vi "Get Protocol Type.vi"(8 "error in (no error)":errorcluster, 11 "RS-xxx to GPIB ConvBox in":refnum<class "RS-xxx to GPIB ConvBox.lvclass">) -> (0 "error out":errorcluster, 2 "Protocol Type":T1=enum."AK RS-XXX", 3 "RS-xxx to GPIB ConvBox out":refnum<class "RS-xxx to GPIB ConvBox.lvclass">)   [LabVIEW 2018, in "Protocols.lvlib" / "RS-xxx to GPIB ConvBox.lvclass"]
doc: "Returns GPIB ConvBox protocol type Enum.\n\nInput:\nRS-xxx to GPIB ConvBox in: represents an instance of the RS-xxx to GPIB ConvBox protocol class.\n\nOutput: \nRS-xxx to GPIB ConvBox out: represents an instance of the RS-xxx to GPIB ConvBox protocol class provided as input.\nProtocol Type: represents the type of the protocol in Enum format."
uses:
  RS-xxx to GPIB ConvBox.lvclass
  Protocol Parent/Types/Protocol Type.ctl
  Protocol Parent/Protocol Parent.lvclass
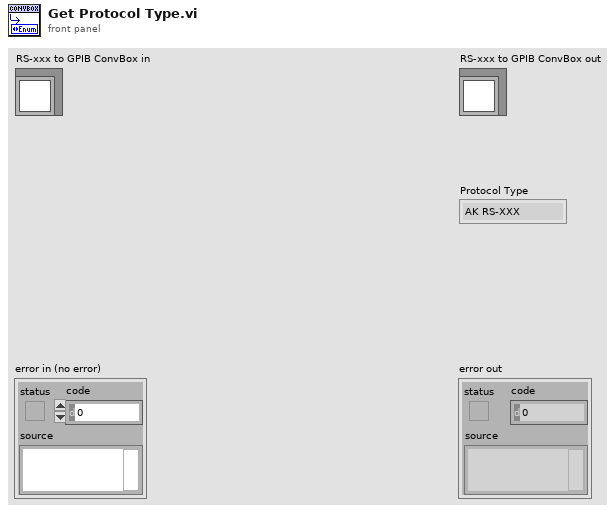
[diagram p1: front panel]
types:
  T1 = typedef "Protocols.lvlib/Protocol Parent.lvclass/Protocol Type.ctl" = enum16{"RS-XXX", "AK RS-XXX", "VISA", "TCPIP", "AK TCPIP", "UDP", "GPIB ConvBox"}
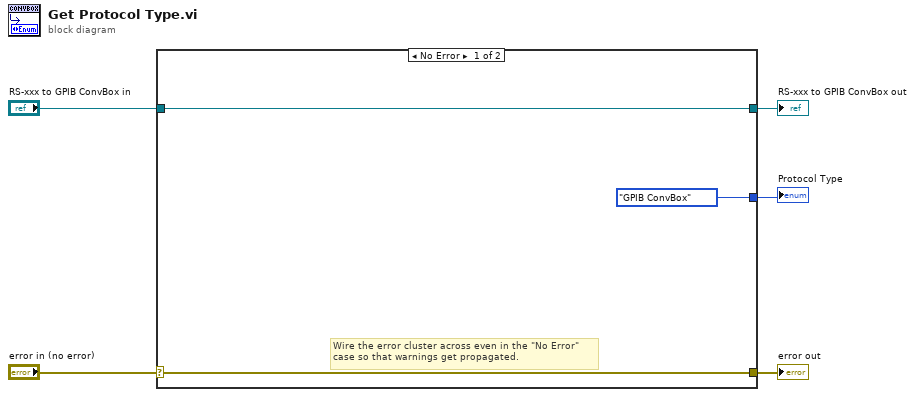
[diagram p0: block diagram]
diagram:
  n1 = case shown="No Error" "error in (no error)" {
    selector: "error in (no error)" -> [w7 w10]
    tunnel: [w7 w10] -> w4
    tunnel: [w8 w9] -> w2
    tunnel: "RS-xxx to GPIB ConvBox in" -> [w8 w9]
    tunnel: [Protocol_Type."GPIB ConvBox" ("Protocol out") _] -> w1
    frame No Error {
      # "Wire the error cluster across even in the \"No Error\"\ncase so that warnings get propagated."
    }
    frame Error {
    }
  }
  "error out" <- w4
  "RS-xxx to GPIB ConvBox out" <- w2
  "Protocol Type" <- w1
